vi "Parse Tokens.vi"(4 "Disable LabVIEW Extensions":bool, 6 "Pretty Print":bool, 10 "Offset":i32, 11 "JSON":string) -> (2 "Tokens":T1[](array[typedef]))   [LabVIEW 2020, in "JSONtext.lvlib"]
uses:
  <vilib>/JDP Science/JSONtext/JSONtext.lvlib
  <vilib>/JDP Science/JSONtext/Parsing/Tokens/Token.ctl
  <vilib>/JDP Science/JSONtext/Parsing/Token Type.ctl
  <vilib>/JDP Science/JSONtext/Parsing/Parsing State.ctl
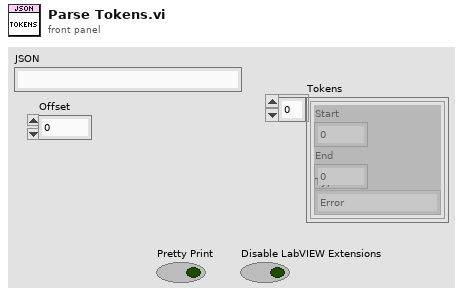
[diagram p1: front panel]
types:
  T1 = typedef "JSONtext.lvlib/Token.ctl" = cluster{"Start":i32, "End":i32, "Type":T2}
  T2 = typedef "JSONtext.lvlib/Token Type.ctl" = enum16{"Error", "Scalar", "comma", "colon", "Comment", "Down", "Up", "Line End", "Make Null", "Inline Comment", "Ignore", "junk line"}
  T3 = typedef "JSONtext.lvlib/Parsing State.ctl" = enum16{"Parser Error", "Object", "Array", "String", "Number/Other", "Leading Whitespace", "Object end", "Array end", "Value end"}
  T4 = cluster{"Offset of first non-whitespace":i32, "Offset past match":i32, T2}
  T5 = cluster{"Offset of first non-whitespace":i32, i32, T2}
  T6 = cluster{"Offset of first non-whitespace":i32, "Offset of first non-whitespace":i32, T2}
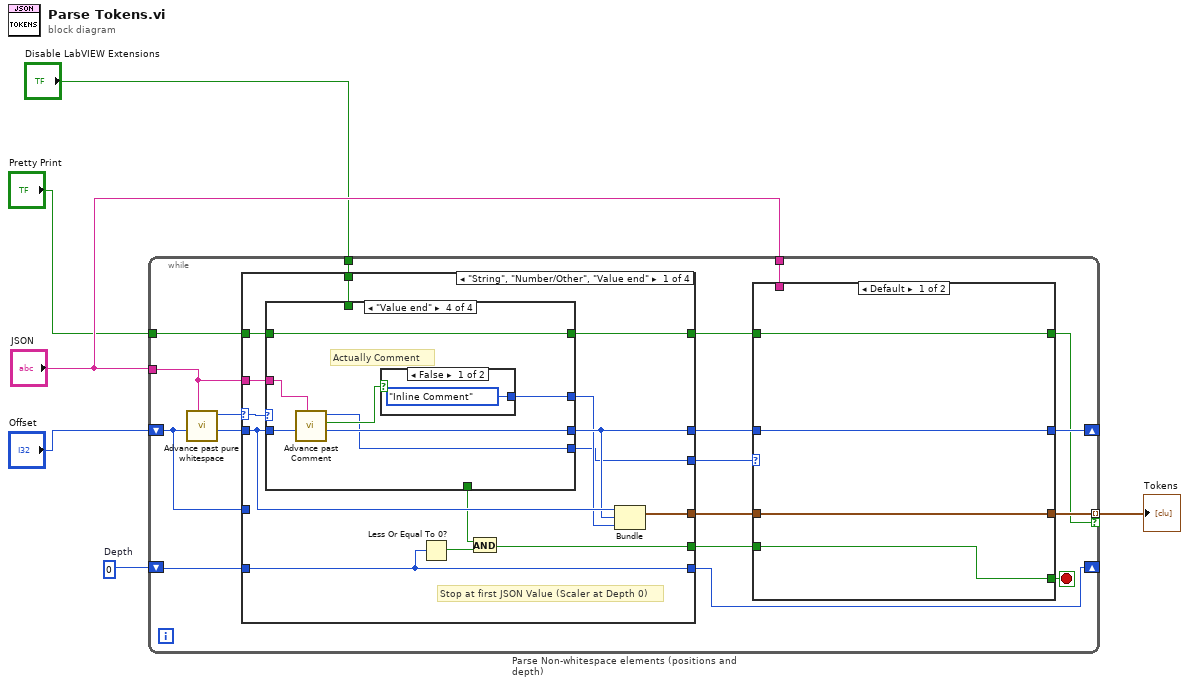
[diagram p0: block diagram]
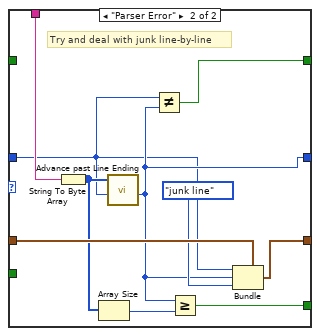
[diagram p2: hidden frame]
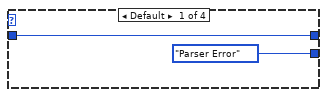
[diagram p3: hidden frame]
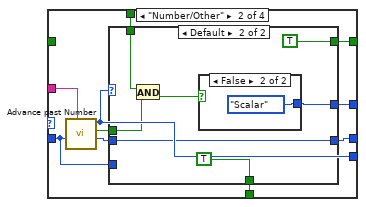
[diagram p4: hidden frame]
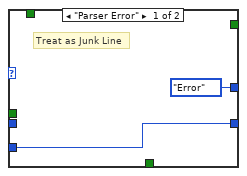
[diagram p5: hidden frame]
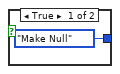
[diagram p6: hidden frame]
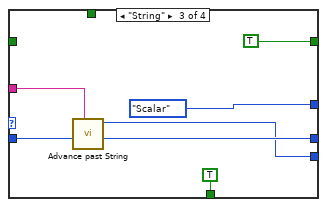
[diagram p7: hidden frame]
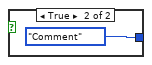
[diagram p8: hidden frame]
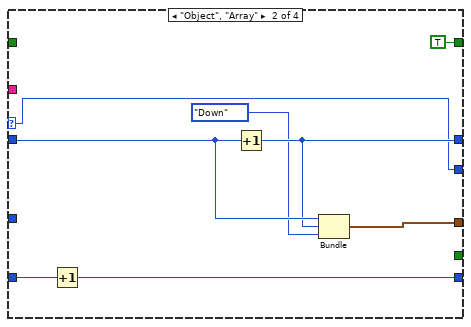
[diagram p9: hidden frame]
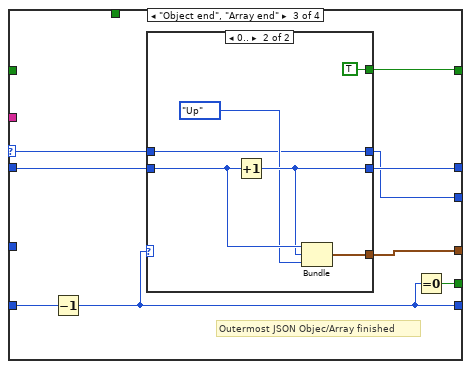
[diagram p10: hidden frame]
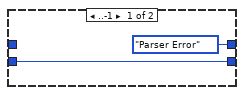
[diagram p11: hidden frame]
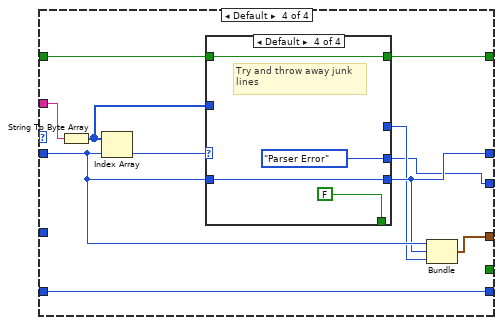
[diagram p12: hidden frame]
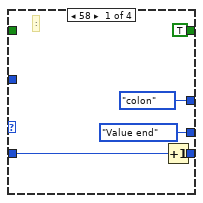
[diagram p13: hidden frame]
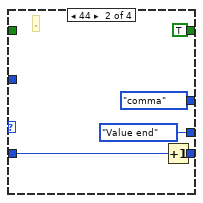
[diagram p14: hidden frame]
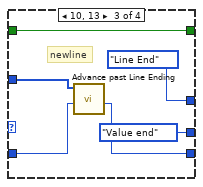
[diagram p15: hidden frame]
diagram:
  w1 = 0  # Depth
  n1 = while "Parse Non-whitespace elements (positions and depth)" {
    tunnel: "JSON" -> [w24]
    shift-right: [w12] -> _
    shift-left: "Offset" -> [w21]
    tunnel: [w15] -> w4 mode=indexing if=w10
    tunnel: "Disable LabVIEW Extensions" -> [w20]
    tunnel: "Pretty Print" -> [w19]
    tunnel: "JSON" -> [w17]
    shift-right: [w8] -> _
    shift-left: w1 -> [w9]
    stop <- w13 stop-if-true
    n2 = call <vilib>:"Advance past pure whitespace.vi"("JSON"=w24, "Offset"=w21) -> ("Offset of first non-whitespace"=w23:i32, "Parser State"=w22:T3)  [unwired: 8 in]
    n3 = case shown="\"String\", \"Number/Other\", \"Value end\"" w22 {
      selector: w22 -> [w51 w94 w104 _]
      tunnel: w24 -> [w52 _ _ w127]
      tunnel: w23 -> [w49 w98 w107 w123]
      tunnel: [w48 w97 w106 w122] -> w18
      tunnel: w21 -> [_ _ _ _]
      tunnel: [w50 w99 w108 w124] -> w16
      tunnel: w20 -> [w47 _ _ _]
      tunnel: w19 -> [w45 _ _ w119]
      tunnel: [w44 TRUE ("Pretty Print") w102 w120] -> w11
      tunnel: [w43 w94 w103 w118] -> w14
      tunnel: w9 -> [w42 w93 w105 w117]
      tunnel: [w42 w92 w101 w117] -> w8
      tunnel: [w39 _ w100 _] -> w7
      frame "String", "Number/Other", "Value end" {
        # "Stop at first JSON Value (Scaler at Depth 0)"
        n4 = case shown="\"Value end\"" w51 {
          tunnel: w52 -> [_ w64 w82 w89]
          tunnel: w49 -> [w54 w56 w81 w88]
          tunnel: [w54 w58 w80 w87] -> w48
          tunnel: [_ w63 Token_Type."Scalar" w86] -> w46
          tunnel: w47 -> [_ w61 _ _]
          tunnel: w45 -> [_ _ _ w84]
          tunnel: [_ w60 TRUE ("Pretty Print") w84] -> w44
          tunnel: [Parsing_State."Parser Error" ("State") w59 w77 w83] -> w43
          tunnel: [_ w55 TRUE _] -> w40
          frame Default {
          }
          frame "Number/Other" {
            n5 = call <vilib>:"Advance past Number.vi"("JSON"=w64, "Offset (0)"=w56) -> ("Offset past match"=w57:i32, "LabVIEW Extension (NaN, Infinity)"=w62:bool, "Parser State"=w59:T3)  [unwired: 5 in, 2 out]
            n6 = case shown="Default" w59 {
              tunnel: [Token_Type."Error" w73] -> w63
              tunnel: w62 -> [_ w72]
              tunnel: w61 -> [_ w70]
              tunnel: [_ TRUE ("Pretty Print")] -> w60
              tunnel: [w66 w68] -> w58
              tunnel: w57 -> [_ w68]
              tunnel: w56 -> [w66 _]
              tunnel: [_ TRUE] -> w55
              frame "Parser Error" {
                # "Treat as Junk Line"
              }
              frame Default {
                n7 = And(x=w70, y=w72) -> (x .and. y?=w71:bool)
                n8 = case shown="False" w71 {
                  tunnel: [Token_Type."Make Null" Token_Type."Scalar"] -> w73
                  frame True {
                  }
                  frame False {
                  }
                }
              }
            }
          }
          frame "String" {
            n9 = call <vilib>:"Advance past String.vi"("JSON"=w82, "Offset"=w81) -> ("Offset past match"=w80:i32, "State"=w77:T3)  [unwired: 7 in, 1 out]
          }
          frame "Value end" {
            # "Actually Comment"
            n10 = call <vilib>:"Advance past Comment.vi"("JSON"=w89, "Offset"=w88) -> ("Offset past match"=w87:i32, "Line End Comment"=w85:bool, "State"=w83:T3)  [unwired: 7 in]
            n11 = case shown="False" w85 {
              tunnel: [Token_Type."Inline Comment" Token_Type."Comment"] -> w86
              frame False {
              }
              frame True {
              }
            }
          }
        }
        n12 = Less Or Equal To 0?(x=w42) -> (x <= 0?=w41:bool)
        n13 = And(x=w40, y=w41) -> (x .and. y?=w39:bool)
        n14 = Bundle("Offset of first non-whitespace"=w49, "Offset past match"=w48, w46) -> (w50:T4)  [unwired: 1 in]
      }
      frame "Object", "Array" {
        n15 = Increment(x=w93) -> (x+1=w92:i32)
        n16 = Increment(x=w98) -> (x+1=w97:i32)
        n17 = Bundle("Offset of first non-whitespace"=w98, w97, Token_Type."Down") -> (w99:T5)  [unwired: 1 in]
      }
      frame "Object end", "Array end" {
        # "Outermost JSON Objec/Array finished"
        n18 = Decrement(x=w105) -> (x-1=w101:i32)
        n19 = case shown="0.." w101 {
          tunnel: [_ w116] -> w108
          tunnel: w107 -> [w109 w115]
          tunnel: [w109 w114] -> w106
          tunnel: w104 -> [_ w112]
          tunnel: [Parsing_State."Parser Error" ("Parser State") w112] -> w103
          tunnel: [_ TRUE ("Pretty Print")] -> w102
          frame ..-1 {
          }
          frame 0.. {
            n20 = Increment(x=w115) -> (x+1=w114:i32)
            n21 = Bundle("Offset of first non-whitespace"=w115, w114, Token_Type."Up") -> (w116:T5)  [unwired: 1 in]
          }
        }
        n22 = Equal To 0?(x=w101) -> (x = 0?=w100:bool)
      }
      frame Default {
        n23 = String To Byte Array(string=w127) -> (unsigned byte array=w125:u8[])
        n24 = Index Array(array=w125, index=w123) -> (element=w126:u8)
        n25 = case shown="Default" w126 {
          tunnel: w125 -> [_ _ w143 _]
          tunnel: w123 -> [w131 w136 w142 w145]
          tunnel: [w132 w137 w141 w145] -> w122
          tunnel: [_ _ _ FALSE] -> _
          tunnel: [Token_Type."colon" Token_Type."comma" Token_Type."Line End" _] -> w121
          tunnel: [TRUE ("Pretty Print") TRUE ("Pretty Print") w139 w146] -> w120
          tunnel: w119 -> [_ _ w139 w146]
          tunnel: [Parsing_State."Value end" ("Parser State") Parsing_State."Value end" ("Parser State") Parsing_State."Value end" ("Parser State") Parsing_State."Parser Error" ("Parser State")] -> w118
          frame 58 {
            # ":"
            n26 = Increment(x=w131) -> (x+1=w132:i32)
          }
          frame 44 {
            # ","
            n27 = Increment(x=w136) -> (x+1=w137:i32)
          }
          frame 10, 13 {
            # "newline"
            n28 = call <vilib>:"Advance past Line Ending.vi"("Offset"=w142, "JSON"=w143) -> ("Offset after Line Ending"=w141:i32)  [unwired: 9 in]
          }
          frame Default {
            # "Try and throw away junk\nlines"
          }
        }
        n29 = Bundle("Offset of first non-whitespace"=w123, "Offset of first non-whitespace"=w122, w121) -> (w124:T6)  [unwired: 1 in]
      }
    }
    n30 = case shown="Default" w14 {
      tunnel: w18 -> [w27 w30]
      tunnel: w17 -> [_ w38]
      tunnel: w16 -> [w28 w37]
      tunnel: [w28 w36] -> w15
      tunnel: [w25 w32] -> w13
      tunnel: [w27 w31] -> w12
      tunnel: w11 -> [w26 _]
      tunnel: [w26 w29] -> w10
      tunnel: w7 -> [w25 _]
      frame Default {
      }
      frame "Parser Error" {
        # "Try and deal with junk line-by-line"
        n31 = String To Byte Array(string=w38) -> (unsigned byte array=w34:u8[])
        n32 = Array Size(array=w34) -> (size(s)=w33:i32)
        n33 = call <vilib>:"Advance past Line Ending.vi"("Offset"=w30, "JSON"=w34) -> ("Offset after Line Ending"=w31:i32)  [unwired: 9 in]
        n34 = Not Equal?(x=w30, y=w31) -> (x != y?=w29:bool)
        n35 = Greater Or Equal?(x=w31, y=w33) -> (x >= y?=w32:bool)
        n36 = Bundle(cluster=w37, "Offset of first non-whitespace"=w30, "Offset of first non-whitespace"=w31, Token_Type."junk line") -> (w36:T6)
      }
    }
  }
  "Tokens" <- w4
